vi "Trim Quotes.vi"(11 "String":string) -> (3 "String without Quotes":string)   [LabVIEW 2015, in "NI_JSON Parsing.lvlib"]
uses:
  NI_JSON Parsing.lvlib
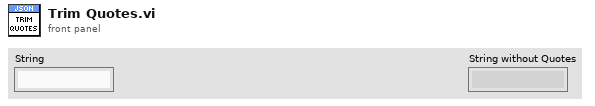
[diagram p1: front panel]
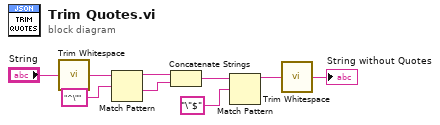
[diagram p0: block diagram]
diagram:
  n1 = call <vilib>:"Trim Whitespace.vi"("string"="String") -> ("trimmed string"=w3:string)  [unwired: 1 in]
  n2 = Match Pattern(string=w3, regular expression="^\"") -> (before substring=w5:string, after substring=w6:string)  [unwired: 1 in, 2 out]
  n3 = Concatenate Strings(w5, w6) -> (w7:string)
  n4 = Match Pattern(string=w7, regular expression="\"$") -> (before substring=w9:string)  [unwired: 1 in, 3 out]
  n5 = call <vilib>:"Trim Whitespace.vi"("string"=w9) -> ("trimmed string"=→"String without Quotes":string)  [unwired: 1 in]
